vi "Interpret INI String.vi"(8 "error in":errorcluster, 10 "INI String":string) -> (0 "error out":errorcluster, 2 "Config Map":variant)   [LabVIEW 2021, in "BS120x Driver.lvlib"]
uses:
  BS120x Driver.lvlib
panel:
  out "INI-Like Data":cluster{"name":string, "kv":string[][]}[](array[cluster])
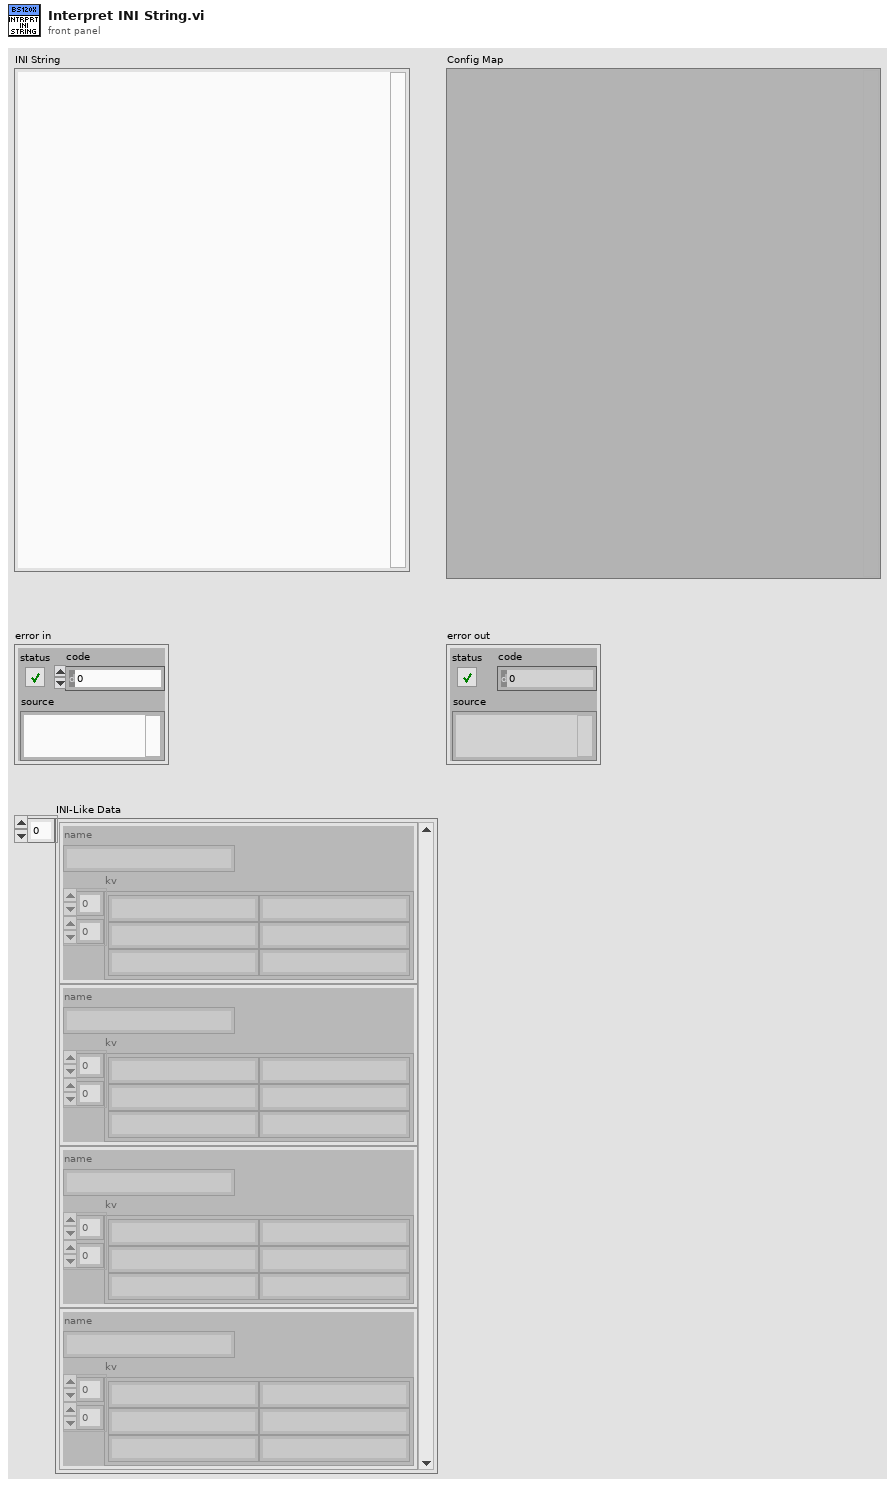
[diagram p1: front panel]
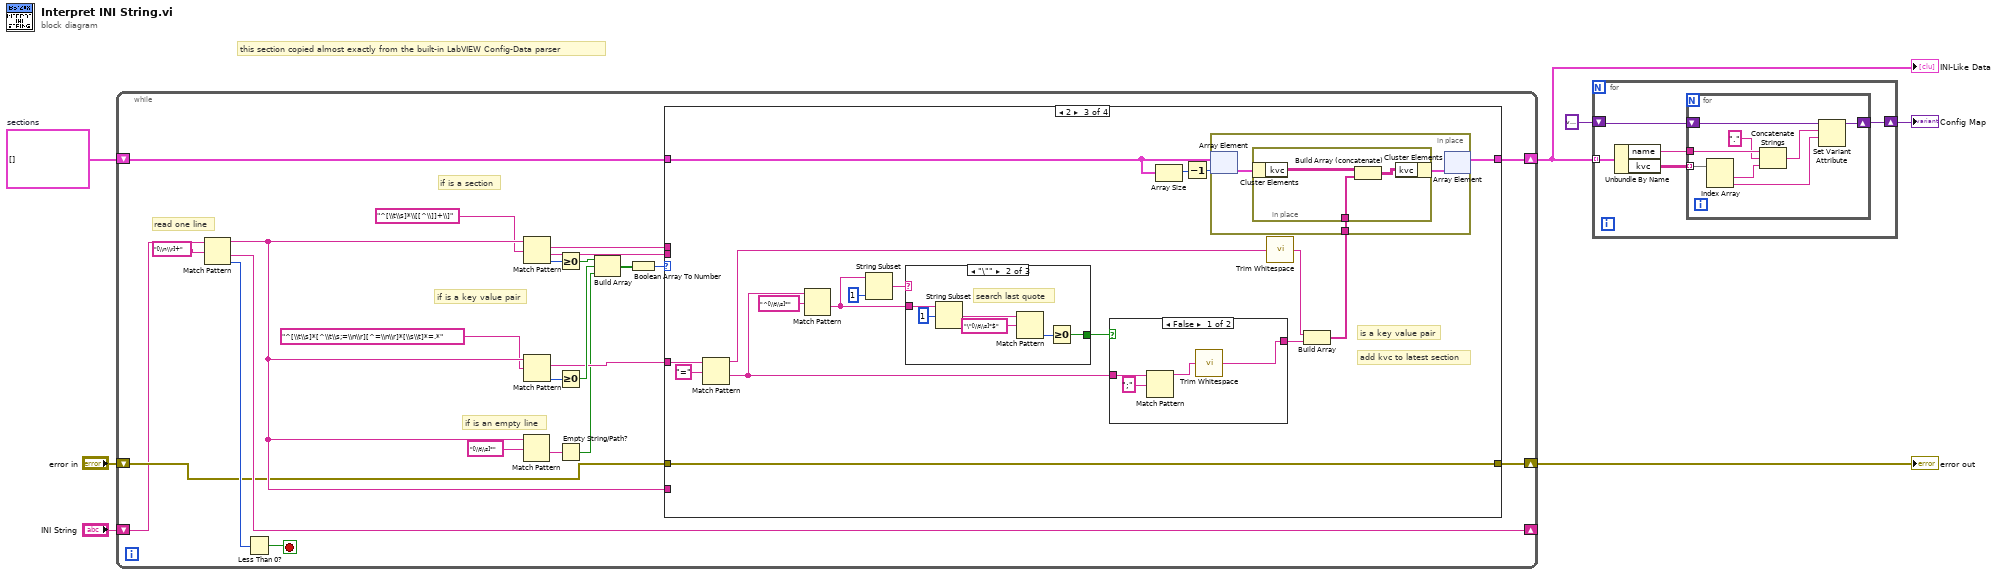
[diagram p0: block diagram]
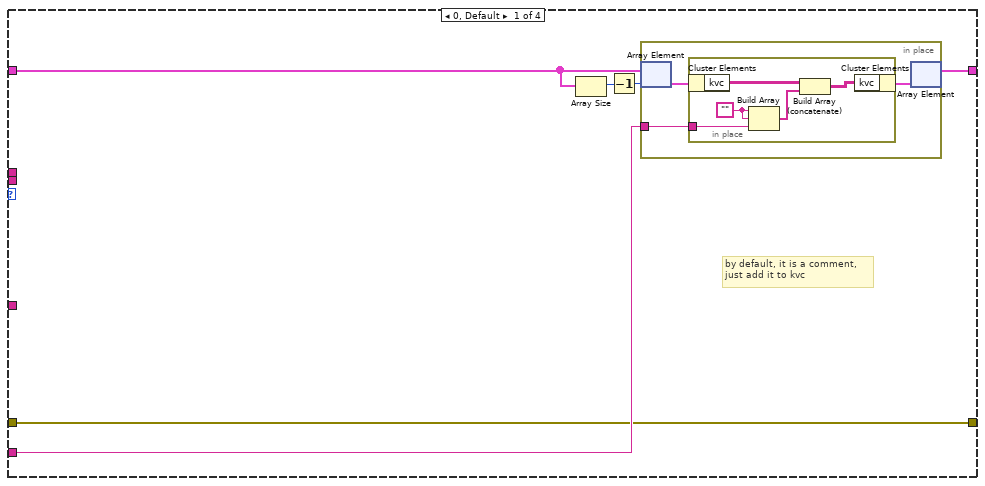
[diagram p2: hidden frame]
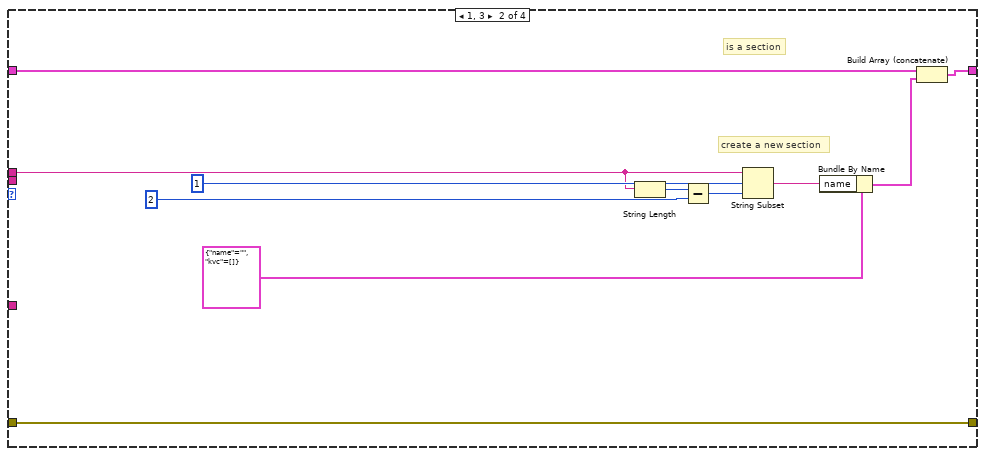
[diagram p3: hidden frame]
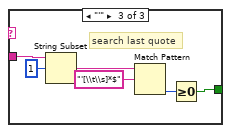
[diagram p5: hidden frame]
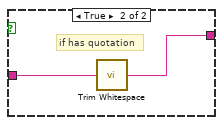
[diagram p6: hidden frame]
diagram:
  w7 = cluster{"name":string, "kvc":string[][]}[] []  # sections
  # "this section copied almost exactly from the built-in LabVIEW Config-Data parser"
  n1 = while {
    shift-right: [w22] -> w2
    shift-left: w7 -> [w23]
    shift-right: [w20] -> w4
    shift-left: "error in" -> [w12]
    shift-right: [w16] -> _
    shift-left: "INI String" -> [w10]
    stop <- w18 stop-if-true
    # "if is an empty line"
    # "if is a key value pair"
    # "if is a section"
    # "read one line"
    n2 = Match Pattern(string=w10, regular expression="[\\n\\r]+") -> (before substring=w14:string, after substring=w16:string, offset past match=w17:i32)  [unwired: 1 in, 1 out]
    n3 = Less Than 0?(x=w17) -> (x < 0?=w18:bool)
    n4 = Match Pattern(string=w14, regular expression="[\\t\\s]*") -> (after substring=w19:string)  [unwired: 1 in, 3 out]
    n5 = Match Pattern(string=w14, regular expression="^[\\t\\s]*\\[[^\\]]+\\]") -> (match substring=w26:string, after substring=w24:string, offset past match=w31:i32)  [unwired: 1 in, 1 out]
    n6 = Match Pattern(string=w14, regular expression="^[\\t\\s]*[^\\t\\s;=\\n\\r][^=\\n\\r]*[\\s\\t]*=.*") -> (match substring=w25:string, offset past match=w11:i32)  [unwired: 1 in, 2 out]
    n7 = Greater Or Equal To 0?(x=w31) -> (x >= 0?=w30:bool)
    n8 = Greater Or Equal To 0?(x=w11) -> (x >= 0?=w29:bool)
    n9 = Empty String/Path?(string/path=w19) -> (empty?=w21:bool)
    n10 = Build Array(w30, w29, w21) -> (w28:bool[])
    n11 = Boolean Array To Number(Boolean array=w28) -> (number=w27:u32)
    n12 = case shown="2" w27 {
      tunnel: w26 -> [_ w46 _ _]
      tunnel: w25 -> [_ _ w64 _]
      tunnel: w14 -> [w34 _ _ _]
      tunnel: w24 -> [_ _ _ _]
      tunnel: w23 -> [w37 w49 w73 w99]
      tunnel: [w33 w48 w70 w99] -> w22
      tunnel: w12 -> [w32 w47 w57 w98]
      tunnel: [w32 w47 w57 w98] -> w20
      frame 0, Default {
        # "by default, it is a comment, \njust add it to kvc"
        n13 = Array Size(array=w37) -> (size(s)=w35:i32)
        n14 = Decrement(x=w35) -> (x-1=w36:i32)
        n15 = in-place {
          in-place-border: w34 -> [w40]
          n16 = in-place-array #1(w37, w36) -> (w39:cluster{"name":string, "kvc":string[][]})
          n17 = in-place {
            in-place-border: w40 -> [w44]
            w45 = ""
            n18 = in-place-cluster #2(w39) -> ("kvc"=w42:string[][])
            n19 = Build Array(w45, w45, w44) -> (w43:string[])
            n20 = Build Array (concatenate)(w42, w43) -> (w41:string[][])
            n21 = in-place-cluster #2("kvc"=w41) -> (w38:cluster{"name":string, "kvc":string[][]})
          }
          n22 = in-place-array #1(w38) -> (w33:cluster{"name":string, "kvc":string[][]}[])  [unwired: 1 out]
        }
      }
      frame 1, 3 {
        # "is a section"
        # "create a new section"
        n23 = String Length(string=w46) -> (length=w54:i32)
        n24 = Subtract(x=w54, y=2) -> (x-y=w55:i32)
        n25 = String Subset(string=w46, offset (0)=1, length (rest)=w55) -> (substring=w51:string)
        n26 = Bundle By Name(cluster=cluster{"name":string, "kvc":string[][]} {"name"="", "kvc"=[]} ("Section"), "name"=w51) -> (w50:cluster{"name":string, "kvc":string[][]})
        n27 = Build Array (concatenate)(w49, w50) -> (w48:cluster{"name":string, "kvc":string[][]}[])
      }
      frame 2 {
        # "is a key value pair"
        # "add kvc to latest section"
        n28 = Match Pattern(string=w64, regular expression="=") -> (before substring=w68:string, after substring=w58:string)  [unwired: 1 in, 2 out]
        n29 = Match Pattern(string=w58, regular expression="^[\\t\\s]*") -> (after substring=w63:string)  [unwired: 1 in, 3 out]
        n30 = String Subset(string=w63, length (rest)=1 ("length (rest)")) -> (substring=w62:string)  [unwired: 1 in]
        n31 = case shown="\"\\\"\"" w62 {
          tunnel: [_ w78 w84] -> w59
          tunnel: w63 -> [_ w76 w82]
          frame Default {
          }
          frame "\"" {
            # "search last quote"
            n32 = String Subset(string=w76, offset (0)=1 ("length (rest)")) -> (substring=w75:string)  [unwired: 1 in]
            n33 = Match Pattern(string=w75, regular expression="\"[\\t\\s]*$") -> (offset past match=w74:i32)  [unwired: 1 in, 3 out]
            n34 = Greater Or Equal To 0?(x=w74) -> (x >= 0?=w78:bool)
          }
          frame "'" {
            # "search last quote"
            n35 = String Subset(string=w82, offset (0)=1 ("length (rest)")) -> (substring=w81:string)  [unwired: 1 in]
            n36 = Match Pattern(string=w81, regular expression="'[\\t\\s]*$") -> (offset past match=w80:i32)  [unwired: 1 in, 3 out]
            n37 = Greater Or Equal To 0?(x=w80) -> (x >= 0?=w84:bool)
          }
        }
        n38 = case shown="False" w59 {
          tunnel: [w86 w91] -> w66
          tunnel: w58 -> [w88 w90]
          frame False {
            n39 = Match Pattern(string=w88, regular expression=";") -> (before substring=w87:string)  [unwired: 1 in, 3 out]
            n40 = call <vilib>:"Trim Whitespace.vi"("string"=w87) -> ("trimmed string"=w86:string)  [unwired: 1 in]
          }
          frame True {
            # "if has quotation"
            n41 = call <vilib>:"Trim Whitespace.vi"("string"=w90) -> ("trimmed string"=w91:string)  [unwired: 1 in]
          }
        }
        n42 = Array Size(array=w73) -> (size(s)=w71:i32)
        n43 = Decrement(x=w71) -> (x-1=w72:i32)
        n44 = call <vilib>:"Trim Whitespace.vi"("string"=w68) -> ("trimmed string"=w67:string)  [unwired: 1 in]
        n45 = Build Array(w67, w66) -> (w65:string[])
        n46 = in-place {
          in-place-border: w65 -> [w92]
          n47 = in-place-array #3(w73, w72) -> (w94:cluster{"name":string, "kvc":string[][]})
          n48 = in-place {
            in-place-border: w92 -> [w95]
            n49 = in-place-cluster #4(w94) -> ("kvc"=w97:string[][])
            n50 = Build Array (concatenate)(w97, w95) -> (w96:string[][])
            n51 = in-place-cluster #4("kvc"=w96) -> (w93:cluster{"name":string, "kvc":string[][]})
          }
          n52 = in-place-array #3(w93) -> (w70:cluster{"name":string, "kvc":string[][]}[])  [unwired: 1 out]
        }
      }
      frame 4 {
        # "empty line"
      }
    }
  }
  "INI-Like Data" <- w2
  "error out" <- w4
  n53 = for {
    tunnel: w2 -> [w104] mode=indexing
    shift-right: [w100] -> w1
    shift-left: variant -> [w102]
    n54 = Unbundle By Name(w104) -> ("name"=w101:string, "kvc"=w103:string[][])
    n55 = for {
      tunnel: w103 -> [w112] mode=indexing
      shift-right: [w109] -> w100
      shift-left: w102 -> [w110]
      tunnel: w101 -> [w108]
      n56 = Index Array(array=w112) -> (element #1=w106:string, element #2=w111:string)  [unwired: 2 in]
      n57 = Concatenate Strings(w108, "." ("name"), w106) -> (w105:string)
      n58 = Set Variant Attribute(Variant=w110, name=w105, value=w111) -> (Variant out=w109:variant)  [unwired: 1 in, 2 out]
    }
  }
  "Config Map" <- w1
